vi "Keithley 2450 Digitized Sweep.vi"() -> ()   [LabVIEW 2020]
doc: "Configure the sweep with the amplitude, source settings and takes current and voltage reading.\n\nNote:\nThis VI is applicable only to 2461 model."
uses:
  <instrlib>/Keithley 2450/Public/Data/Read (Multiple Points).vi
  <instrlib>/Keithley 2450/Keithley 2450.lvlib
panel:
  in  "Digital Voltage Range (1.0)":dbl=0.1
  in  "Digital Current Range (1.0)":dbl=0.1
  in  "Limit Level (0.1)":dbl=0.1
  in  "Delay (0) in Sec":dbl
  in  "Sample Rate (1000Hz)":u32=2500
  in  "Sweep Points":T1={"Start "=0.0, "Stop "=5.0, "Number of Points (5)"=100}
  in  "Source Mode  (0: Voltage)":u16(ring) items=["Voltage", "Current"]
  in  "VISA resource name":refnum<visa-resource-name>
  out "Waveform Graph":dbl[][](graph)=[[-0.0001858189, 0.007417283, 0.03360542, 0.04403445, 0.04793108, 0.04931186, 0.04991157, 0.05009001, 0.050169, 0.05021289, 0.05022166, 0.0502948, 0.05017778, 0.0501924, 0.05012805, 0.05020703, 0.05027724, 0.05013097, 0.05005784, 0.05013682, 0.05028309, 0.05022166, 0.05016023, 0.05013682, 0.05026846, 0.05003736, 0.05026846, 0.05008124, 0.04967754, 0.06964044, 0.08971742, 0.09662428, 0.09915767, 0.1002605, 0.1006028, 0.1006964, 0.1009071, 0.1008047, 0.1007023, 0.1006935, 0.10079, 0.1007959, 0.1007725, 0.1007988, 0.100673, 0.1007198, 0.1008105, 0.1007052, 0.1007257, 0.1006584, 0.1006935, 0.1007754, 0.1007754, 0.1007637, 0.1007052, 0.1005882, 0.1131528, 0.1376734, 0.146435, 0.1495388, 0.1505656, 0.1511127, 0.1512063, 0.1512092, 0.1511624, 0.151139, 0.1511624, 0.1513233, 0.1511917, 0.1512999, 0.1512005, 0.151256, 0.1513321, 0.1512209, 0.1512239, 0.1510981, 0.1511624, 0.1513233, 0.1512472, 0.1512999, 0.1512999, 0.1513496, 0.151256, 0.1512999, 0.1734568, 0.1922818, 0.1985187, 0.2007771, 0.2015465, 0.2017893, 0.2019765, 0.2018595, 0.201842, 0.2017601, 0.2017893, 0.2019063, 0.2018215, 0.2016898, 0.2017103, 0.2018069], [-0.0001858189, 0.007417283, 0.03360542, 0.04403445, 0.04793108, 0.04931186, 0.04991157, 0.05009001, 0.050169, 0.05021289, 0.05022166, 0.0502948, 0.05017778, 0.0501924, 0.05012805, 0.05020703, 0.05027724, 0.05013097, 0.05005784, 0.05013682, 0.05028309, 0.05022166, 0.05016023, 0.05013682, 0.05026846, 0.05003736, 0.05026846, 0.05008124, 0.04967754, 0.06964044, 0.08971742, 0.09662428, 0.09915767, 0.1002605, 0.1006028, 0.1006964, 0.1009071, 0.1008047, 0.1007023, 0.1006935, 0.10079, 0.1007959, 0.1007725, 0.1007988, 0.100673, 0.1007198, 0.1008105, 0.1007052, 0.1007257, 0.1006584, 0.1006935, 0.1007754, 0.1007754, 0.1007637, 0.1007052, 0.1005882, 0.1131528, 0.1376734, 0.146435, 0.1495388, 0.1505656, 0.1511127, 0.1512063, 0.1512092, 0.1511624, 0.151139, 0.1511624, 0.1513233, 0.1511917, 0.1512999, 0.1512005, 0.151256, 0.1513321, 0.1512209, 0.1512239, 0.1510981, 0.1511624, 0.1513233, 0.1512472, 0.1512999, 0.1512999, 0.1513496, 0.151256, 0.1512999, 0.1734568, 0.1922818, 0.1985187, 0.2007771, 0.2015465, 0.2017893, 0.2019765, 0.2018595, 0.201842, 0.2017601, 0.2017893, 0.2019063, 0.2018215, 0.2016898, 0.2017103, 0.2018069]]
  # "(c) 2021 National Instruments.  ALL RIGHTS RESERVED."
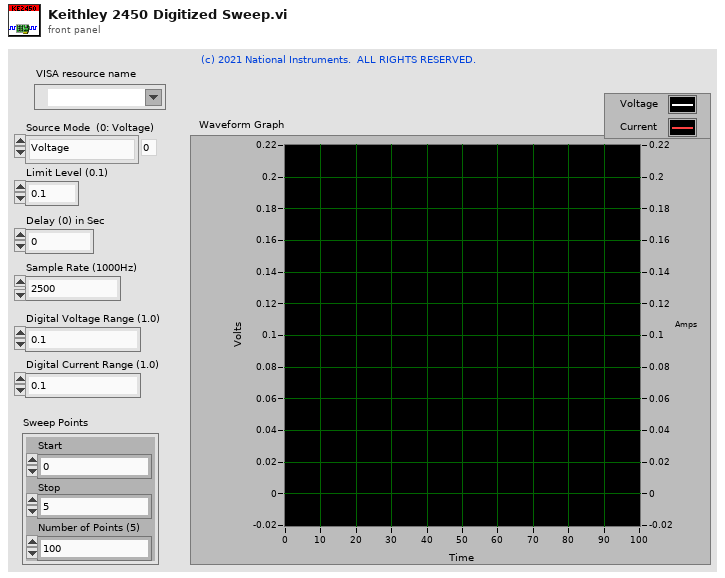
[diagram p1: front panel]
types:
  T1 = cluster{"Start ":dbl, "Stop ":dbl, "Number of Points (5)":u32}
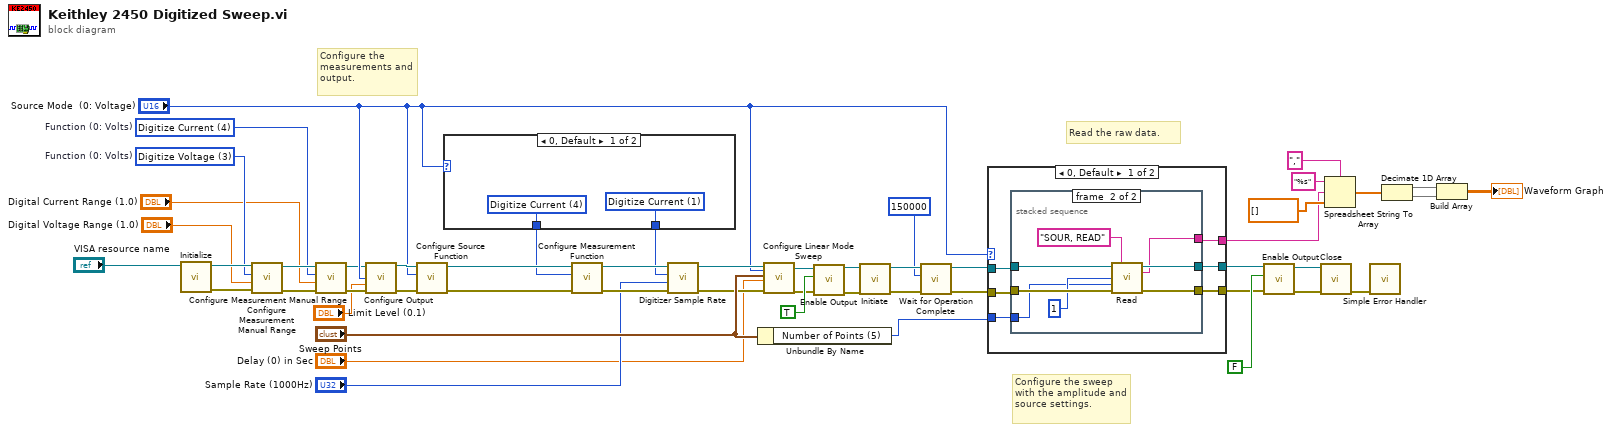
[diagram p0: block diagram]
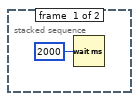
[diagram p2: hidden frame]
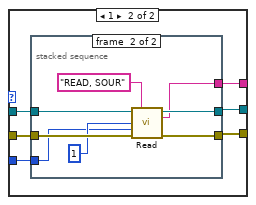
[diagram p3: hidden frame]
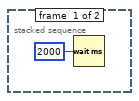
[diagram p4: hidden frame]
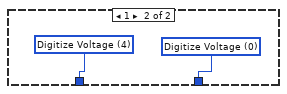
[diagram p5: hidden frame]
diagram:
  w8 = u16 4 items=["Volts", "Current", "Resistance", "Digitize Voltage", "Digitize Current"]  # Function (0: Volts)
  w9 = u16 3 items=["Volts", "Current", "Resistance", "Digitize Voltage", "Digitize Current"]  # Function (0: Volts)
  # "Read the raw data."
  # "Configure the sweep with the amplitude and source settings."
  # "Configure the measurements and output."
  n1 = call <instrlib>:"Initialize.vi"("VISA resource name"="VISA resource name") -> ("error out"=w14:errorcluster, "VISA resource name out"=w15:refnum<visa-resource-name>)  [unwired: 9 in]
  n2 = call <instrlib>:"Configure Measurement Manual Range.vi"("error in (no error)"=w14, "Manual Range (1.0)"="Digital Voltage Range (1.0)", "Function (0: Volts)"=w9, "VISA resource name"=w15) -> ("error out"=w12:errorcluster, "VISA resource name out"=w13:refnum<visa-resource-name>)  [unwired: 6 in]
  n3 = call <instrlib>:"Configure Measurement Manual Range.vi"("error in (no error)"=w12, "Manual Range (1.0)"="Digital Current Range (1.0)", "Function (0: Volts)"=w8, "VISA resource name"=w13) -> ("error out"=w10:errorcluster, "VISA resource name out"=w11:refnum<visa-resource-name>)  [unwired: 6 in]
  n4 = call <instrlib>:"Configure Output.vi"("VISA resource name"=w11, "Source Mode  (0: Voltage)"="Source Mode  (0: Voltage)", "Source Limit Level (0.1)"="Limit Level (0.1)", "error in (no error)"=w10) -> ("VISA resource name out"=w44:refnum<visa-resource-name>, "error out"=w45:errorcluster)  [unwired: 10 in]
  n5 = call <instrlib>:"Configure Source Function.vi"("error in (no error)"=w45, "Function (0: Volts)"="Source Mode  (0: Voltage)", "VISA resource name"=w44) -> ("error out"=w27:errorcluster, "VISA resource name out"=w28:refnum<visa-resource-name>)  [unwired: 7 in]
  n6 = case shown="0, Default" "Source Mode  (0: Voltage)" {
    tunnel: [w53 w55] -> w7
    tunnel: [w52 w54] -> w6
    frame 0, Default {
      w52 = u16 1 items=["Digitize Voltage", "Digitize Current"] ("Function (0: Volts)")
      w53 = u16 4 items=["Voltage", "Current", "Resistance", "Digitize Voltage", "Digitize Current"] ("Function (0: Volts)")
    }
    frame 1 {
      w54 = u16 0 items=["Digitize Voltage", "Digitize Current"] ("Function (0: Volts)")
      w55 = u16 4 items=["Voltage", "Current", "Auto Resistance", "Manual Resistance", "Digitize Voltage", "Digitize Current"] ("Function (0: Volts)")
    }
  }
  n7 = call <instrlib>:"Configure Measurement Function.vi"("error in (no error)"=w27, "Function (0: Volts)"=w7, "VISA resource name"=w28) -> ("error out"=w19:errorcluster, "VISA resource name out"=w20:refnum<visa-resource-name>)  [unwired: 7 in]
  n8 = call <instrlib>:"Digitizer Sample Rate.vi"("error in (no error)"=w19, "Sample Rate (100000)"="Sample Rate (1000Hz)", "Digitize Function (Voltage)"=w6, "VISA resource name"=w20) -> ("error out"=w17:errorcluster, "VISA resource name out"=w18:refnum<visa-resource-name>)  [unwired: 6 in]
  n9 = Unbundle By Name("Sweep Points") -> ("Number of Points (5)"=w22:u32)
  n10 = call <instrlib>:"Configure Linear Mode Sweep.vi"("VISA resource name"=w18, "Source Mode  (0: Voltage)"="Source Mode  (0: Voltage)", "Sweep Points"="Sweep Points", "Delay (0)"="Delay (0) in Sec", "error in (no error)"=w17) -> ("VISA resource name out"=w43:refnum<visa-resource-name>, "error out"=w42:errorcluster)  [unwired: 13 in]
  n11 = call <instrlib>:"Enable Output.vi"("error in (no error)"=w42, "Enable Output (T: Enable)"=TRUE, "VISA resource name"=w43) -> ("error out"=w40:errorcluster, "VISA resource name out"=w41:refnum<visa-resource-name>)  [unwired: 7 in]
  n12 = call <instrlib>:"Initiate.vi"("error in (no error)"=w40, "VISA resource name"=w41) -> ("error out"=w30:errorcluster, "VISA resource name out"=w31:refnum<visa-resource-name>)  [unwired: 8 in]
  n13 = call <instrlib>:"Wait for Operation Complete.vi"("error in (no error)"=w30, "Timeout (10000 ms)"=150000, "VISA resource name"=w31) -> ("error out"=w25:errorcluster, "VISA resource name out"=w26:refnum<visa-resource-name>)  [unwired: 7 in]
  n14 = case shown="0, Default" "Source Mode  (0: Voltage)" {
    tunnel: w26 -> [w61 w76]
    tunnel: w25 -> [w60 w75]
    tunnel: [w59 w73] -> w24
    tunnel: [w58 w72] -> w23
    tunnel: w22 -> [w57 w74]
    tunnel: [w56 w71] -> w21
    frame 0, Default {
      n15 = stacked-sequence {
        tunnel: [_ w70] -> w59
        tunnel: [_ w69] -> w58
        tunnel: w61 -> [_ w67]
        tunnel: w60 -> [_ w66]
        tunnel: [_ w65] -> w56
        tunnel: w57 -> [_ w63]
        frame #0 {
          n16 = Wait (ms)(milliseconds to wait=u32 2000) -> ()  [unwired: 1 out]
        }
        frame #1 {
          n17 = call-poly <instrlib>:"Read.vi"("VISA resource name"=w67, "Buffer Elements"="SOUR, READ", "Start Index (1)"=1, "End Index (1)"=w63, "error in (no error)"=w66) -> ("VISA resource name out"=w70:refnum<visa-resource-name>, "Data out"=w65:string, "error out"=w69:errorcluster)  [unwired: 8 in]
        }
      }
    }
    frame 1 {
      n18 = stacked-sequence {
        tunnel: [_ w85] -> w73
        tunnel: [_ w84] -> w72
        tunnel: w76 -> [_ w82]
        tunnel: w75 -> [_ w81]
        tunnel: [_ w80] -> w71
        tunnel: w74 -> [_ w78]
        frame #0 {
          n19 = Wait (ms)(milliseconds to wait=u32 2000) -> ()  [unwired: 1 out]
        }
        frame #1 {
          n20 = call-poly <instrlib>:"Read.vi"("VISA resource name"=w82, "Buffer Elements"="READ, SOUR", "Start Index (1)"=1, "End Index (1)"=w78, "error in (no error)"=w81) -> ("VISA resource name out"=w85:refnum<visa-resource-name>, "Data out"=w80:string, "error out"=w84:errorcluster)  [unwired: 8 in]
        }
      }
    }
  }
  n21 = call <instrlib>:"Enable Output.vi"("error in (no error)"=w23, "Enable Output (T: Enable)"=FALSE, "VISA resource name"=w24) -> ("error out"=w48:errorcluster, "VISA resource name out"=w49:refnum<visa-resource-name>)  [unwired: 7 in]
  n22 = call <instrlib>:"Close.vi"("error in (no error)"=w48, "VISA resource name"=w49) -> ("error out"=w50:errorcluster)  [unwired: 9 in]
  n23 = Spreadsheet String To Array(delimiter (Tab)=",", format string="%s", spreadsheet string=w21, array type (2D Dbl)=dbl[] []) -> (array=w35:dbl[])
  n24 = call <vilib>:"Simple Error Handler.vi"("error in (no error)"=w50) -> ()  [unwired: 4 in, 5 out]
  n25 = Decimate 1D Array(w35) -> (w34:dbl[], w33:dbl[])
  n26 = Build Array(w34, w33) -> (→"Waveform Graph":dbl[][])
